vi "ParserScales.vi"(8 "error in (no error)":errorcluster, 11 "JSON item":string) -> (0 "error out":errorcluster, 2 "scales":T1[](array[typedef]), 3 "JSON item":string)   [LabVIEW 2017, in "Paser.lvlib"]
uses:
  Paser.lvlib
  <vilib>/JDP Science/JSONtext/JSONtext.lvlib
  Ctrl/ScaleType.ctl
  Ctrl/Scale.ctl
  Ctrl/TableScale.ctl
  00ce7b0f-547f-47ea-b810-7f5e95fdae9d.vi
  Ctrl/PolynomialScale.ctl
  34cb3f1a-c200-4327-976c-325a63f53796.vi
  Ctrl/LinearScale.ctl
  5c05d997-d596-41e5-b13d-dcf8b246c8cd.vi
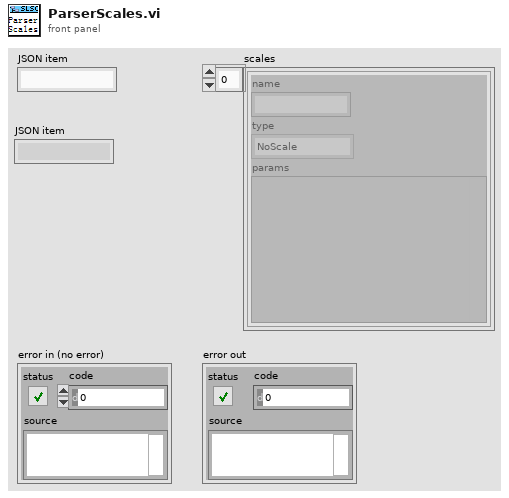
[diagram p1: front panel]
types:
  T1 = typedef "Scale.ctl" = cluster{"name":string, "type":T2, "params":variant}
  T2 = typedef "ScaleType.ctl" = enum16{"NoScale", "Table", "Polynomial", "Linear"}
  T3 = typedef "TableScale.ctl" = cluster{"name":string, "coercion":string, "table":cluster{"scaled":dbl, "unscaled":dbl}[]}
  T4 = typedef "PolynomialScale.ctl" = cluster{"name":string, "forwardCoeffs":dbl[], "reverseCoeffs":dbl[]}
  T5 = typedef "LinearScale.ctl" = cluster{"name":string, "m":dbl, "b":dbl}
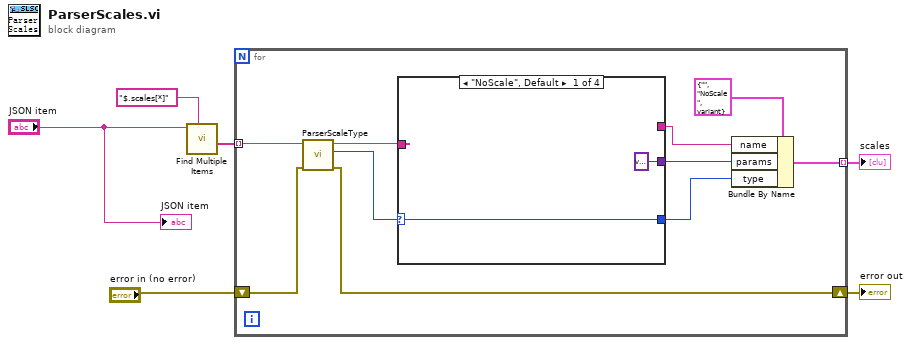
[diagram p0: block diagram]
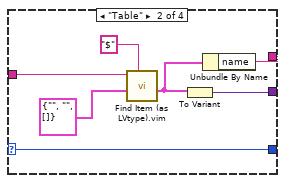
[diagram p2: hidden frame]
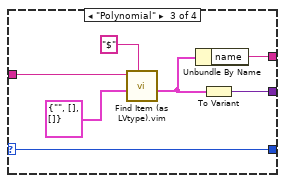
[diagram p3: hidden frame]
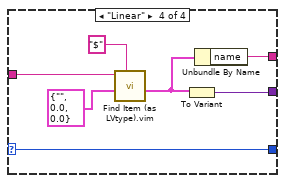
[diagram p4: hidden frame]
diagram:
  n1 = call <vilib>:"Find Multiple Items.vi"("$Path or Item Name"="$.scales[*]", "JSON"="JSON item") -> ("<JSON>"=w3:string[])  [unwired: 6 in, 3 out]
  n2 = for {
    tunnel: w3 -> [w16] mode=indexing
    shift-right: [w8] -> w5
    shift-left: "error in (no error)" -> [w9]
    tunnel: [w7] -> w6 mode=indexing
    n3 = call "ParserScaleType.vi"("error in (no error)"=w9, "JSON item"=w16) -> ("error out"=w8:errorcluster, "Scale Type"=w15:T2, "JSON item"=w14:string)  [unwired: 7 in]
    n4 = case shown="\"NoScale\", Default" w15 {
      selector: w15 -> [w17 w19 w27 w33]
      tunnel: w14 -> [_ w24 w31 w39]
      tunnel: [variant ("Variant") w20 w28 w34] -> w12
      tunnel: [w17 w19 w27 w33] -> w11
      tunnel: [_ w21 w26 w35] -> w13
      frame "NoScale", Default {
      }
      frame "Table" {
        n5 = call "Find Item (as LVtype).vim"("$Path or Item Name"="$", "Data Type and Default Value"=T3 {"name"="", "coercion"="", "table"=[]}, "JSON"=w24) -> ("Data"=w22:T3)  [unwired: 5 in, 3 out]
        n6 = To Variant(anything=w22) -> (Variant=w20:variant)
        n7 = Unbundle By Name(w22) -> ("name"=w21:string)
      }
      frame "Polynomial" {
        n8 = call "Find Item (as LVtype).vim"("$Path or Item Name"="$", "Data Type and Default Value"=T4 {"name"="", "forwardCoeffs"=[], "reverseCoeffs"=[]} ("PolynomialScale"), "JSON"=w31) -> ("Data"=w29:T4)  [unwired: 5 in, 3 out]
        n9 = Unbundle By Name(w29) -> ("name"=w26:string)
        n10 = To Variant(anything=w29) -> (Variant=w28:variant)
      }
      frame "Linear" {
        n11 = call "Find Item (as LVtype).vim"("$Path or Item Name"="$", "Data Type and Default Value"=T5 {"name"="", "m"=0.0, "b"=0.0} ("linear"), "JSON"=w39) -> ("Data"=w36:T5)  [unwired: 5 in, 3 out]
        n12 = To Variant(anything=w36) -> (Variant=w34:variant)
        n13 = Unbundle By Name(w36) -> ("name"=w35:string)
      }
    }
    n14 = Bundle By Name(cluster=T1 {"name"="", "type"=enum."NoScale", "params"=variant}, "name"=w13, "params"=w12, "type"=w11) -> (w7:T1)
  }
  "error out" <- w5
  "scales" <- w6
  "JSON item" <- "JSON item"
